vi "Begin.vi"(11 "Image Size":T1=enum."160x120") -> (0 "error out":errorcluster)   [LabVIEW 2011]
doc: "Called before other user functions, this VI is expected to open initial I/O refnums, load in file data, and do all program initialization. Notice that the <B>error out</B> terminal is simply used for data flow. Wiring it to other structures or subVIs ensures that this VI runs first."
uses:
  <vilib>/Rock Robotics/WPI/Camera/WPI_CameraImageSize.ctl
  <vilib>/Rock Robotics/WPI/Camera/WPI_CameraWhite Balance Values.ctl
  <vilib>/Rock Robotics/WPI/Camera/WPI_CameraExposure Values.ctl
  <vilib>/Rock Robotics/WPI/Camera/WPI_CameraFrameRate.ctl
  <vilib>/Rock Robotics/SystemInterfaces/DIO/FPGA_DIOPWMChannel.ctl
  <vilib>/Rock Robotics/SystemInterfaces/Typedef/FPGA_TypedefDigitalModule.ctl
  <vilib>/Rock Robotics/SystemInterfaces/Typedef/FPGA_TypedefAnalogModule.ctl
  <vilib>/Rock Robotics/SystemInterfaces/AI/FPGA_AIChannel.ctl
  <vilib>/Rock Robotics/SystemInterfaces/DIO/FPGA_DIOChannel.ctl
  <vilib>/Rock Robotics/SystemInterfaces/DIO/FPGA_DIORelayChannel.ctl
  <vilib>/Rock Robotics/WPI/Joystick/WPI_JoystickDeviceEnum.ctl
  <vilib>/Rock Robotics/WPI/Relay/WPI_RelayDirection.ctl
  <vilib>/Rock Robotics/SystemInterfaces/Typedef/FPGA_TypedefSolenoidModule.ctl
  <vilib>/Rock Robotics/WPI/Solenoid/WPI_SolenoidChannel.ctl
  <vilib>/Rock Robotics/WPI/RobotDrive/WPI_RobotDriveOpen4MotorWithVictor.vi
  <vilib>/Rock Robotics/WPI/MotorControl/WPI_MotorControlOpen Victor.vi
  <vilib>/Rock Robotics/WPI/Counter/WPI_CounterDigitalInputToDigitalSource.vi
  <vilib>/Rock Robotics/WPI/Counter/WPI_CounterOpen Gear Tooth Sensor Mode.vi
  <vilib>/Rock Robotics/WPI/Solenoid/WPI_SolenoidOpenDouble.vi
  <vilib>/Rock Robotics/WPI/Compressor/WPI_CompressorGetSetRefNum.vi
  <vilib>/Rock Robotics/WPI/Encoder/WPI_EncoderType.ctl
panel:
  in  "Image Size 2":T1=enum."160x120"
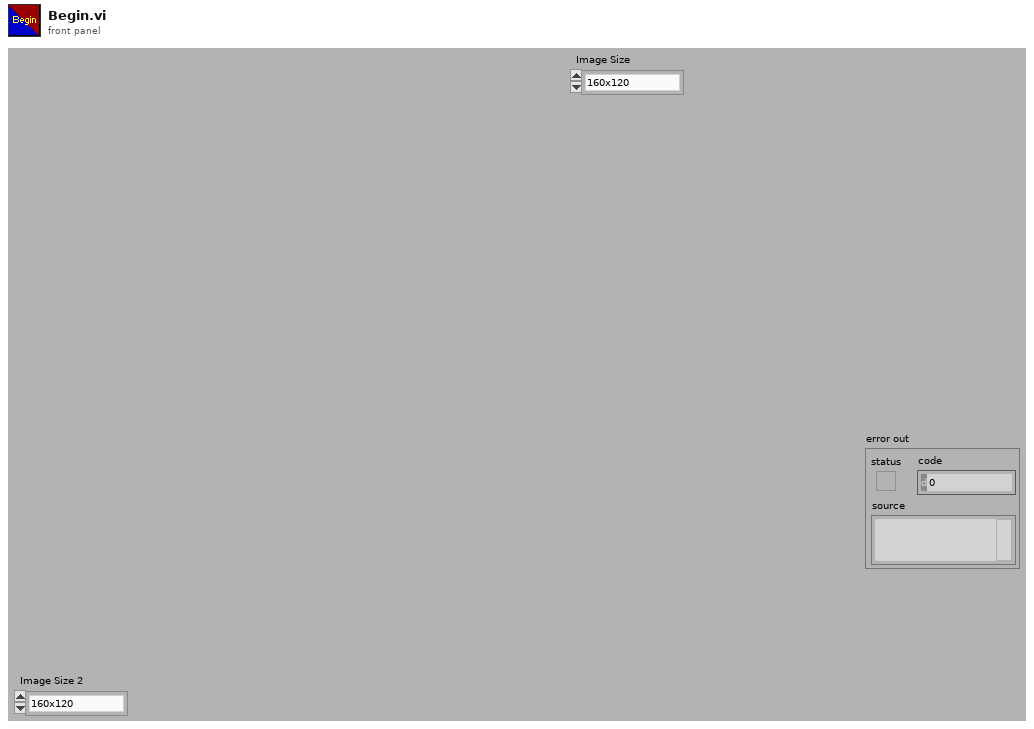
[diagram p1: front panel]
types:
  T1 = typedef "WPI_CameraImageSize.ctl" = enum16{"640x480", "320x240", "160x120"}
  T2 = typedef "FPGA_DIOChannel.ctl" = enum8{"DIO 1", "DIO 2", "DIO 3", "DIO 4", "DIO 5", "DIO 6", "DIO 7", "DIO 8", "DIO 9", "DIO 10", "DIO 11", "DIO 12", "DIO 13", "DIO 14", "Invalid"}
  T3 = typedef "FPGA_TypedefDigitalModule.ctl" = enum16{"Digital Module 1", "Digital Module 2"}
  T4 = typedef "WPI_SolenoidChannel.ctl" = enum8{"Solenoid 1", "Solenoid 2", "Solenoid 3", "Solenoid 4", "Solenoid 5", "Solenoid 6", "Solenoid 7", "Solenoid 8", "Invalid"}
  T5 = typedef "FPGA_TypedefSolenoidModule.ctl" = enum16{"Solenoid Module 1", "Solenoid Module 2"}
  T6 = typedef "WPI_RelayDirection.ctl" = enum16{"Both directions", "Forward only", "Reverse only"}
  T7 = typedef "FPGA_DIORelayChannel.ctl" = enum8{"Relay 1", "Relay 2", "Relay 3", "Relay 4", "Relay 5", "Relay 6", "Relay 7", "Relay 8", "Invalid"}
  T8 = typedef "WPI_JoystickDeviceEnum.ctl" = enum16{"USB 1", "USB 2", "USB 3", "USB 4", "Kinect 1", "Kinect 2"}
  T9 = typedef "FPGA_DIOPWMChannel.ctl" = enum8{"PWM 1", "PWM 2", "PWM 3", "PWM 4", "PWM 5", "PWM 6", "PWM 7", "PWM 8", "PWM 9", "PWM 10", "Invalid"}
  T10 = typedef "FPGA_AIChannel.ctl" = enum8{"AI 1", "AI 2", "AI 3", "AI 4", "AI 5", "AI 6", "AI 7", "AI 8", "Invalid"}
  T11 = typedef "FPGA_TypedefAnalogModule.ctl" = enum16{"Analog Module 1", "Analog Module 2"}
  T12 = typedef "WPI_CameraFrameRate.ctl" = u32
  T13 = typedef "WPI_CameraExposure Values.ctl" = enum16{"Auto", "Flicker-free 50 Hz", "Flicker-free 60 Hz", "Hold current"}
  T14 = typedef "WPI_CameraWhite Balance Values.ctl" = enum16{"Auto", "Fixed indoor", "Fixed outdoor 1", "Fixed outdoor 2", "Fixed fluorescent 1", "Fixed fluorescent 2", "Hold current"}
  T15 = typedef "WPI_MotorControlDeviceRef.ctl" = cluster{"DeviceStatus":errorcluster, "Type":enum16{"PWM", "CAN"}, "PWM":cluster{"Digital Module":T3, "PWM Channel":T9, "DeadBand":T16}, "CAN":cluster{"Device Number":u8, "Control Mode":T17, "Semaphore":T18, "Max Vout":dbl}, "Invert":bool, "TransformRef":T19, "InvTransformRef":T19}
  T16 = typedef "WPI_PWMDeadband.ctl" = cluster{"Name":string, "maxPositivePwm":i32, "minPositivePwm":i32, "centerPwm":i32, "maxNegativePwm":i32, "minNegativePwm":i32, "angularRange":u16}
  T17 = typedef "WPI_CANJaguar_ControlMode.ctl" = enum8{"Percent VBus", "Current", "Speed", "Position", "Voltage"}
  T18 = typedef "Semaphore RefNum" = refnum<k1>
  T19 = typedef "WPI_PWMTransform_ConPane.ctl" = refnum<vi>
  T20 = typedef "WPI_RobotDriveDevRef.ctl" = cluster{"DevStatus":errorcluster, "Motors[]":T15[], "Square Inputs":bool, "Max Output":dbl, "Isochronous":bool}
  T21 = typedef "WPI_CameraDevRef.ctl" = cluster{"Camera Address":string, "CameraStatus":errorcluster, "Acquire Image Notifier":refnum<notifier>}
  T22 = typedef "WPI_EncoderType.ctl" = enum16{"1x", "2x", "4x"}
  T23 = typedef "WPI_DigitalInputDevRef.ctl" = cluster{"DevStatus":errorcluster, "DIO Channel":T2, "Digital Module":T3}
  T24 = typedef "FPGA_CounterEncoderSourceConvertionLVSourceType.ctl" = cluster{"DevStatus":errorcluster, "AnalogTriggerMode?":bool, "DigitalMode":cluster{"Digital Module":T3, "DIO Channel":T25}, "AnalogTriggerMode":cluster{"AnalogTriggerIndex":T26, "OutputType":T27}}
  T25 = typedef "FPGA_DIODigitalSourceChannel.ctl" = enum8{"DIO 1", "DIO 2", "DIO 3", "DIO 4", "DIO 5", "DIO 6", "DIO 7", "DIO 8", "DIO 9", "DIO 10", "DIO 11", "DIO 12", "DIO 13", "DIO 14", "Disabled"}
  T26 = typedef "FPGA_AnalogTriggerIndex.ctl" = enum8{"Trig 0", "Trig 1", "Trig 2", "Trig 3", "Trig 4", "Trig 5", "Trig 6", "Trig 7", "Invalid"}
  T27 = typedef "FPGA_AnalogTriggerOutType.ctl" = enum16{"InWindow", "TriggerState", "Rising", "Falling"}
  T28 = typedef "WPI_EncoderDevRef.ctl" = cluster{"DevStatus":errorcluster, "EncoderIndex":T29, "CounterIndex":T30, "DistancePerCount":dbl, "Decoding Type":T22}
  T29 = typedef "FPGA_EncoderIdx.ctl" = enum8{"Enc 0", "Enc 1", "Enc 2", "Enc 3", "Invalid"}
  T30 = typedef "FPGA_CounterCtrSystemIndex.ctl" = enum8{"Ctr 0", "Ctr 1", "Ctr 2", "Ctr 3", "Ctr 4", "Ctr 5", "Ctr 6", "Ctr 7", "Invalid"}
  T31 = typedef "WPI_JoystickDevRef.ctl" = cluster{"Device":T8}
  T32 = typedef "WPI_AnalogChannelDevRef.ctl" = cluster{"DevStatus":errorcluster, "Analog Module":T11, "Analog Channel":T10}
  T33 = typedef "WPI_RelayDevRef.ctl" = cluster{"DevStatus":errorcluster, "Relay Channel":T7, "Digital Module":T3, "Relay Direction":T6}
  T34 = typedef "WPI_SolenoidDevRef.ctl" = cluster{"DevStatus":errorcluster, "Solenoid Module":T5, "Forward Solenoid Channel":T4, "Reverse Solenoid Channel":T4}
  T35 = typedef "WPI_CompressorDevRef.ctl" = cluster{"DevStatus":errorcluster, "DigitalInputDevRef":T23, "RelayDevRef":T33}
  T36 = typedef "WPI_CounterDevRef.ctl" = cluster{"DevStatus":errorcluster, "CntIndex":T30}
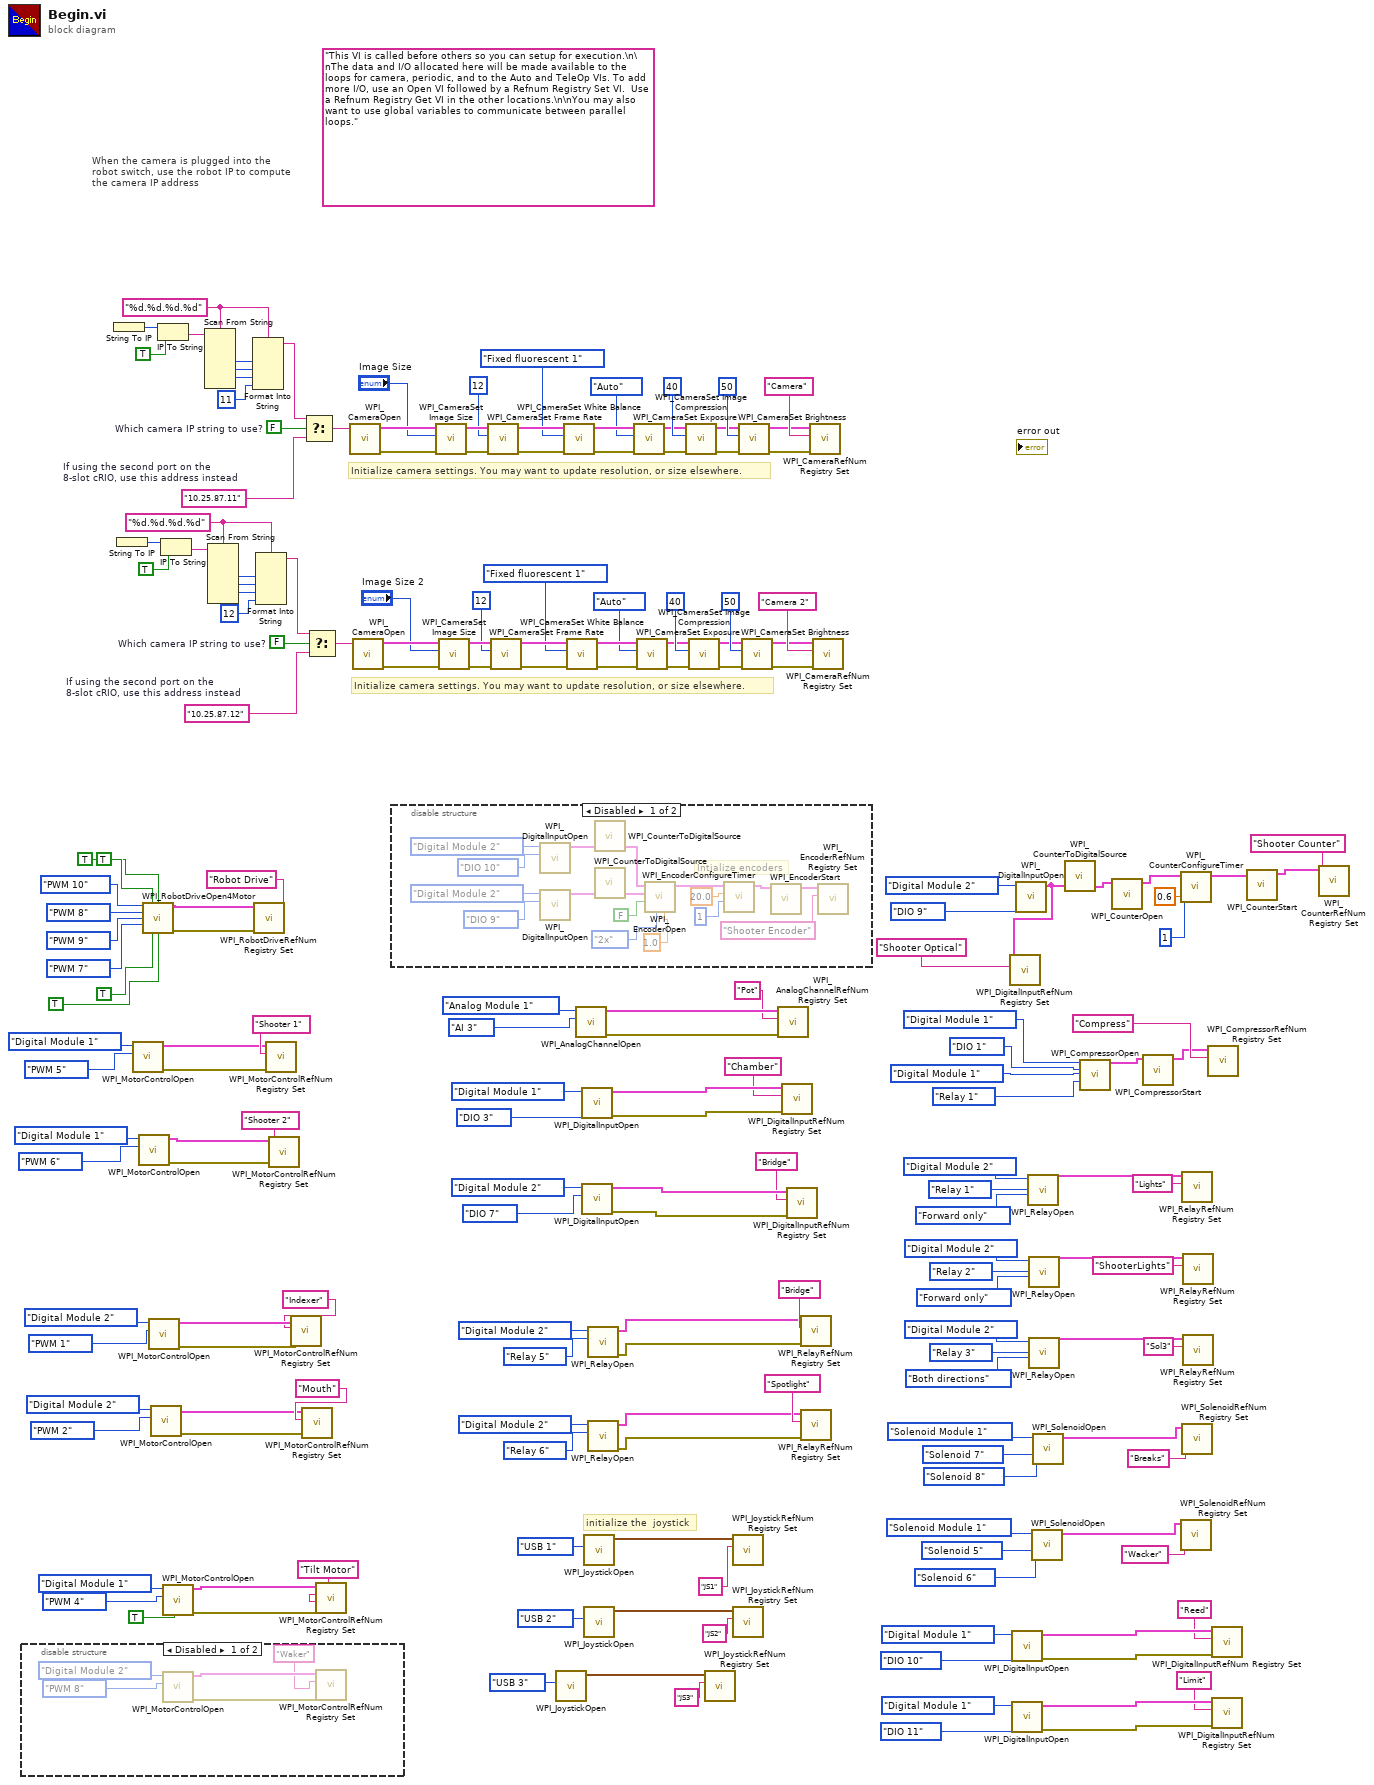
[diagram p0: block diagram]
diagram:
  w125 = FALSE  # Which camera IP string to use?
  w129 = "%d.%d.%d.%d" ("format string")
  w126 = "10.25.87.12"  # If using the second port on the 8-slot cRIO, use this address instead
  w158 = FALSE  # Which camera IP string to use?
  w162 = "%d.%d.%d.%d" ("format string")
  (unwired) "This VI is called before others so you can setup for execution.\n\nThe data and I/O allocated here will be made available to the loops for camera, periodic, and to the Auto and TeleOp VIs. To add more I/O, use an Open VI followed by a Refnum Registry Set VI.  Use a Refnum Registry Get VI in the other locations.\n\nYou may also want to use global variables to communicate between parallel loops."
  w159 = "10.25.87.11"  # If using the second port on the 8-slot cRIO, use this address instead
  # "initialize the  joystick"
  # "Initialize camera settings. You may want to update resolution, or size elsewhere."
  # "When the camera is plugged into the\nrobot switch, use the robot IP to compute\nthe camera IP address"
  # "Initialize camera settings. You may want to update resolution, or size elsewhere."
  n1 = disable-structure shown="Disabled" {
    frame Disabled {
      n2 = call-poly <vilib>:"WPI_MotorControlOpen.vi"("PWM Channel"=FPGA_DIOPWMChannel."PWM 8", "Digital Module (Module 1)"=FPGA_TypedefDigitalModule."Digital Module 2") -> ("error out"=w195:errorcluster, "MotorControlDeviceRef"=w194:T15)  [unwired: 8 in]
      n3 = call <vilib>:"WPI_MotorControlRefNum Registry Set.vi"("error in (no error)"=w195, "refnum name"="Waker", "MotorControlDevRef"=w194) -> ()  [unwired: 7 in, 2 out]
    }
    frame Enabled {
    }
  }
  n4 = String To IP() -> (0:w169:u32)  [unwired: 1 in]
  n5 = String To IP() -> (0:w136:u32)  [unwired: 1 in]
  n6 = call-poly <vilib>:"WPI_MotorControlOpen.vi"("PWM Channel"=FPGA_DIOPWMChannel."PWM 5", "Digital Module (Module 1)"=FPGA_TypedefDigitalModule."Digital Module 1") -> ("error out"=w108:errorcluster, "MotorControlDeviceRef"=w109:T15)  [unwired: 8 in]
  n7 = call-poly <vilib>:"WPI_MotorControlOpen.vi"("PWM Channel"=FPGA_DIOPWMChannel."PWM 6", "Digital Module (Module 1)"=FPGA_TypedefDigitalModule."Digital Module 1") -> ("error out"=w106:errorcluster, "MotorControlDeviceRef"=w107:T15)  [unwired: 8 in]
  n8 = call-poly <vilib>:"WPI_RobotDriveOpen4Motor.vi"("Rear Left Motor"=FPGA_DIOPWMChannel."PWM 10", "Rear Left Motor Inverted"=TRUE, "Rear Right Motor Inverted"=TRUE, "Rear Right Motor"=FPGA_DIOPWMChannel."PWM 8", "Front Left Motor"=FPGA_DIOPWMChannel."PWM 9", "Front Right Motor"=FPGA_DIOPWMChannel."PWM 7", "Front Left Motor Inverted"=TRUE, "Front Right Motor Inverted"=TRUE) -> ("RobotDriveDevRef"=w68:T20, "error out"=w67:errorcluster)  [unwired: 6 in]
  n9 = call-poly <vilib>:"WPI_MotorControlOpen.vi"("PWM Channel"=FPGA_DIOPWMChannel."PWM 1", "Digital Module (Module 1)"=FPGA_TypedefDigitalModule."Digital Module 2") -> ("error out"=w76:errorcluster, "MotorControlDeviceRef"=w77:T15)  [unwired: 8 in]
  n10 = call-poly <vilib>:"WPI_MotorControlOpen.vi"("PWM Channel"=FPGA_DIOPWMChannel."PWM 2", "Digital Module (Module 1)"=FPGA_TypedefDigitalModule."Digital Module 2") -> ("error out"=w101:errorcluster, "MotorControlDeviceRef"=w102:T15)  [unwired: 8 in]
  n11 = IP To String(1:TRUE ("dot notation? (F)"), 2:w169) -> (0:w167:string)
  n12 = IP To String(1:TRUE ("dot notation? (F)"), 2:w136) -> (0:w134:string)
  n13 = call-poly <vilib>:"WPI_MotorControlOpen.vi"("Invert"=TRUE, "PWM Channel"=FPGA_DIOPWMChannel."PWM 4", "Digital Module (Module 1)"=FPGA_TypedefDigitalModule."Digital Module 1") -> ("error out"=w95:errorcluster, "MotorControlDeviceRef"=w96:T15)  [unwired: 7 in]
  n14 = Scan From String(format string=w162, input string=w167) -> (output 1=w166:i32, output 2=w165:i32, output 3=w164:i32)  [unwired: 7 in, 3 out]
  n15 = Scan From String(format string=w129, input string=w134) -> (output 1=w133:i32, output 2=w132:i32, output 3=w131:i32)  [unwired: 7 in, 3 out]
  n16 = Format Into String(format string=w162, w166, w165, w164, 11 ("Compression")) -> (resulting string=w160:string)  [unwired: 2 in, 1 out]
  n17 = call <vilib>:"WPI_RobotDriveRefNum Registry Set.vi"("error in (no error)"=w67, "refnum name"="Robot Drive", "RobotDriveDevRef"=w68) -> ()  [unwired: 7 in, 2 out]
  n18 = Format Into String(format string=w129, w133, w132, w131, 12 ("Compression")) -> (resulting string=w127:string)  [unwired: 2 in, 1 out]
  n19 = call <vilib>:"WPI_MotorControlRefNum Registry Set.vi"("error in (no error)"=w108, "refnum name"="Shooter 1", "MotorControlDevRef"=w109) -> ()  [unwired: 7 in, 2 out]
  n20 = call <vilib>:"WPI_MotorControlRefNum Registry Set.vi"("error in (no error)"=w106, "refnum name"="Shooter 2", "MotorControlDevRef"=w107) -> ()  [unwired: 7 in, 2 out]
  n21 = call <vilib>:"WPI_MotorControlRefNum Registry Set.vi"("error in (no error)"=w76, "refnum name"="Indexer", "MotorControlDevRef"=w77) -> ()  [unwired: 7 in, 2 out]
  n22 = call <vilib>:"WPI_MotorControlRefNum Registry Set.vi"("error in (no error)"=w101, "refnum name"="Mouth", "MotorControlDevRef"=w102) -> ()  [unwired: 7 in, 2 out]
  n23 = Select(t=w160, s=w158, f=w159) -> (s? t:f=w161:string)
  n24 = Select(t=w127, s=w125, f=w126) -> (s? t:f=w128:string)
  n25 = call <vilib>:"WPI_MotorControlRefNum Registry Set.vi"("error in (no error)"=w95, "refnum name"="Tilt Motor", "MotorControlDevRef"=w96) -> ()  [unwired: 7 in, 2 out]
  n26 = call <vilib>:"WPI_CameraOpen.vi"("Camera Address"=w161) -> ("error out"=w181:errorcluster, "CameraDevRef"=w182:T21)  [unwired: 1 in, 8 out]
  n27 = call <vilib>:"WPI_CameraOpen.vi"("Camera Address"=w128) -> ("error out"=w148:errorcluster, "CameraDevRef"=w149:T21)  [unwired: 1 in, 8 out]
  n28 = disable-structure shown="Disabled" {
    frame Disabled {
      # "Intialize encoders"
      n29 = call <vilib>:"WPI_DigitalInputOpen.vi"("DIO Channel"=FPGA_DIOChannel."DIO 10", "Digital Module (Module 1)"=FPGA_TypedefDigitalModule."Digital Module 2") -> ("DigitalInputDevRef"=w210:T23)  [unwired: 8 in, 1 out]
      n30 = call <vilib>:"WPI_DigitalInputOpen.vi"("DIO Channel"=FPGA_DIOChannel."DIO 9", "Digital Module (Module 1)"=FPGA_TypedefDigitalModule."Digital Module 2") -> ("DigitalInputDevRef"=w206:T23)  [unwired: 8 in, 1 out]
      n31 = call-poly <vilib>:"WPI_CounterToDigitalSource.vi"("DigitalInputDevRef"=w210) -> ("Digital Source"=w209:T24)  [unwired: 6 in]
      n32 = call-poly <vilib>:"WPI_CounterToDigitalSource.vi"("DigitalInputDevRef"=w206) -> ("Digital Source"=w205:T24)  [unwired: 6 in]
      n33 = call <vilib>:"WPI_EncoderOpen.vi"("DistancePerCount"=1.0, "Decoding Type"=WPI_EncoderType."2x", "Invert Direction (False)"=FALSE, "BSource"=w205, "ASource"=w209) -> ("EncoderDevRef"=w203:T28)  [unwired: 5 in, 1 out]
      n34 = call <vilib>:"WPI_EncoderConfigureTimer.vi"("Number Samples to Average"=u8 1, "Minimum Rate"=20.0, "EncoderDevRef"=w203) -> ("EncoderDevRef"=w197:T28)  [unwired: 7 in, 1 out]
      n35 = call <vilib>:"WPI_EncoderStart.vi"("EncoderDevRef"=w197) -> ("EncoderDevRef"=w196:T28)  [unwired: 9 in, 1 out]
      n36 = call <vilib>:"WPI_EncoderRefNum Registry Set.vi"("refnum name"="Shooter Encoder", "EncoderDevRef"=w196) -> ()  [unwired: 8 in, 2 out]
    }
    frame Enabled {
    }
  }
  n37 = call <vilib>:"WPI_CameraSet Image Size.vi"("error in (no error)"=w181, "Image Size"="Image Size", "CameraDevRef"=w182) -> ("error out"=w180:errorcluster, "CameraDevRef Out"=w183:T21)  [unwired: 7 out]
  n38 = call <vilib>:"WPI_CameraSet Image Size.vi"("error in (no error)"=w148, "Image Size"="Image Size 2", "CameraDevRef"=w149) -> ("error out"=w147:errorcluster, "CameraDevRef Out"=w150:T21)  [unwired: 7 out]
  n39 = call <vilib>:"WPI_CameraSet Frame Rate.vi"("error in (no error)"=w180, "Frame Rate (fps)"=T12 12, "CameraDevRef"=w183) -> ("error out"=w179:errorcluster, "CameraDevRef Out"=w185:T21)  [unwired: 7 out]
  n40 = call <vilib>:"WPI_CameraSet Frame Rate.vi"("error in (no error)"=w147, "Frame Rate (fps)"=T12 12, "CameraDevRef"=w150) -> ("error out"=w146:errorcluster, "CameraDevRef Out"=w152:T21)  [unwired: 7 out]
  n41 = call <vilib>:"WPI_JoystickOpen.vi"("JoystickDevice"=WPI_JoystickDeviceEnum."USB 3") -> ("JoystickDevRef"=w45:T31)  [unwired: 10 out]
  n42 = call <vilib>:"WPI_CameraSet White Balance.vi"("error in (no error)"=w179, "White Balance"=WPI_CameraWhite_Balance_Values."Fixed fluorescent 1", "CameraDevRef"=w185) -> ("error out"=w178:errorcluster, "CameraDevRef Out"=w184:T21)  [unwired: 7 out]
  n43 = call <vilib>:"WPI_CameraSet White Balance.vi"("error in (no error)"=w146, "White Balance"=WPI_CameraWhite_Balance_Values."Fixed fluorescent 1", "CameraDevRef"=w152) -> ("error out"=w145:errorcluster, "CameraDevRef Out"=w151:T21)  [unwired: 7 out]
  n44 = call <vilib>:"WPI_AnalogChannelOpen.vi"("Analog Channel"=FPGA_AIChannel."AI 3", "Analog Module (Module 1)"=FPGA_TypedefAnalogModule."Analog Module 1") -> ("error out"=w90:errorcluster, "AIDeviceRef"=w92:T32)  [unwired: 8 in]
  n45 = call <vilib>:"WPI_DigitalInputOpen.vi"("DIO Channel"=FPGA_DIOChannel."DIO 3", "Digital Module (Module 1)"=FPGA_TypedefDigitalModule."Digital Module 1") -> ("error out"=w85:errorcluster, "DigitalInputDevRef"=w87:T23)  [unwired: 8 in]
  n46 = call <vilib>:"WPI_DigitalInputOpen.vi"("DIO Channel"=FPGA_DIOChannel."DIO 7", "Digital Module (Module 1)"=FPGA_TypedefDigitalModule."Digital Module 2") -> ("error out"=w57:errorcluster, "DigitalInputDevRef"=w59:T23)  [unwired: 8 in]
  n47 = call <vilib>:"WPI_JoystickOpen.vi"("JoystickDevice"=WPI_JoystickDeviceEnum."USB 1") -> ("JoystickDevRef"=w72:T31)  [unwired: 10 out]
  n48 = call <vilib>:"WPI_JoystickOpen.vi"("JoystickDevice"=WPI_JoystickDeviceEnum."USB 2") -> ("JoystickDevRef"=w71:T31)  [unwired: 10 out]
  n49 = call <vilib>:"WPI_RelayOpen.vi"("Relay Channel"=FPGA_DIORelayChannel."Relay 5", "Digital Module (Module 1)"=FPGA_TypedefDigitalModule."Digital Module 2") -> ("error out"=w62:errorcluster, "RelayDevRef"=w63:T33)  [unwired: 8 in]
  n50 = call <vilib>:"WPI_RelayOpen.vi"("Relay Channel"=FPGA_DIORelayChannel."Relay 6", "Digital Module (Module 1)"=FPGA_TypedefDigitalModule."Digital Module 2") -> ("error out"=w80:errorcluster, "RelayDevRef"=w81:T33)  [unwired: 8 in]
  n51 = call <vilib>:"WPI_CameraSet Exposure.vi"("error in (no error)"=w178, "Exposure"=WPI_CameraExposure_Values."Auto", "CameraDevRef"=w184) -> ("error out"=w177:errorcluster, "CameraDevRef Out"=w187:T21)  [unwired: 7 out]
  n52 = call <vilib>:"WPI_CameraSet Exposure.vi"("error in (no error)"=w145, "Exposure"=WPI_CameraExposure_Values."Auto", "CameraDevRef"=w151) -> ("error out"=w144:errorcluster, "CameraDevRef Out"=w154:T21)  [unwired: 7 out]
  n53 = call <vilib>:"WPI_CameraSet Image Compression.vi"("error in (no error)"=w177, "Compression"=40, "CameraDevRef"=w187) -> ("error out"=w176:errorcluster, "CameraDevRef Out"=w186:T21)  [unwired: 7 out]
  n54 = call <vilib>:"WPI_CameraSet Image Compression.vi"("error in (no error)"=w144, "Compression"=40, "CameraDevRef"=w154) -> ("error out"=w143:errorcluster, "CameraDevRef Out"=w153:T21)  [unwired: 7 out]
  n55 = call <vilib>:"WPI_JoystickRefNum Registry Set.vi"("refnum name"="JS3", "JoystickDevRef"=w45) -> ()  [unwired: 1 in, 9 out]
  n56 = call <vilib>:"WPI_JoystickRefNum Registry Set.vi"("refnum name"="JS1", "JoystickDevRef"=w72) -> ()  [unwired: 1 in, 9 out]
  n57 = call <vilib>:"WPI_JoystickRefNum Registry Set.vi"("refnum name"="JS2", "JoystickDevRef"=w71) -> ()  [unwired: 1 in, 9 out]
  n58 = call <vilib>:"WPI_CameraSet Brightness.vi"("error in (no error)"=w176, "Brightness"=50, "CameraDevRef"=w186) -> ("error out"=w174:errorcluster, "CameraDevRef Out"=w175:T21)  [unwired: 7 out]
  n59 = call <vilib>:"WPI_CameraSet Brightness.vi"("error in (no error)"=w143, "Brightness"=50, "CameraDevRef"=w153) -> ("error out"=w141:errorcluster, "CameraDevRef Out"=w142:T21)  [unwired: 7 out]
  n60 = call <vilib>:"WPI_AnalogChannelRefNum Registry Set.vi"("error in (no error)"=w90, "refnum name"="Pot", "AIDeviceRef"=w92) -> ()  [unwired: 7 in, 2 out]
  n61 = call <vilib>:"WPI_DigitalInputRefNum Registry Set.vi"("error in (no error)"=w85, "refnum name"="Chamber", "DigitalInputDevRef"=w87) -> ()  [unwired: 7 in, 2 out]
  n62 = call <vilib>:"WPI_DigitalInputRefNum Registry Set.vi"("error in (no error)"=w57, "refnum name"="Bridge", "DigitalInputDevRef"=w59) -> ()  [unwired: 7 in, 2 out]
  n63 = call <vilib>:"WPI_RelayRefNum Registry Set.vi"("error in (no error)"=w62, "refnum name"="Bridge", "RelayDevRef"=w63) -> ()  [unwired: 7 in, 2 out]
  n64 = call <vilib>:"WPI_RelayRefNum Registry Set.vi"("error in (no error)"=w80, "refnum name"="Spotlight", "RelayDevRef"=w81) -> ()  [unwired: 7 in, 2 out]
  n65 = call <vilib>:"WPI_CameraRefNum Registry Set.vi"("error in (no error)"=w174, "refnum name"="Camera", "CameraDevRef"=w175) -> ()  [unwired: 9 out]
  n66 = call <vilib>:"WPI_CameraRefNum Registry Set.vi"("error in (no error)"=w141, "refnum name"="Camera 2", "CameraDevRef"=w142) -> ()  [unwired: 9 out]
  n67 = call <vilib>:"WPI_DigitalInputOpen.vi"("DIO Channel"=FPGA_DIOChannel."DIO 10", "Digital Module (Module 1)"=FPGA_TypedefDigitalModule."Digital Module 1") -> ("error out"=w6:errorcluster, "DigitalInputDevRef"=w8:T23)  [unwired: 8 in]
  n68 = call <vilib>:"WPI_DigitalInputOpen.vi"("DIO Channel"=FPGA_DIOChannel."DIO 11", "Digital Module (Module 1)"=FPGA_TypedefDigitalModule."Digital Module 1") -> ("error out"=w1:errorcluster, "DigitalInputDevRef"=w3:T23)  [unwired: 8 in]
  n69 = call <vilib>:"WPI_DigitalInputOpen.vi"("DIO Channel"=FPGA_DIOChannel."DIO 9", "Digital Module (Module 1)"=FPGA_TypedefDigitalModule."Digital Module 2") -> ("DigitalInputDevRef"=w53:T23)  [unwired: 8 in, 1 out]
  n70 = call <vilib>:"WPI_DigitalInputRefNum Registry Set.vi"("refnum name"="Shooter Optical", "DigitalInputDevRef"=w53) -> ()  [unwired: 8 in, 2 out]
  n71 = call <vilib>:"WPI_RelayOpen.vi"("Relay Direction"=WPI_RelayDirection."Forward only", "Relay Channel"=FPGA_DIORelayChannel."Relay 1", "Digital Module (Module 1)"=FPGA_TypedefDigitalModule."Digital Module 2") -> ("RelayDevRef"=w37:T33)  [unwired: 7 in, 1 out]
  n72 = call <vilib>:"WPI_RelayOpen.vi"("Relay Direction"=WPI_RelayDirection."Forward only", "Relay Channel"=FPGA_DIORelayChannel."Relay 2", "Digital Module (Module 1)"=FPGA_TypedefDigitalModule."Digital Module 2") -> ("RelayDevRef"=w32:T33)  [unwired: 7 in, 1 out]
  n73 = call <vilib>:"WPI_RelayOpen.vi"("Relay Direction"=WPI_RelayDirection."Both directions", "Relay Channel"=FPGA_DIORelayChannel."Relay 3", "Digital Module (Module 1)"=FPGA_TypedefDigitalModule."Digital Module 2") -> ("RelayDevRef"=w27:T33)  [unwired: 7 in, 1 out]
  n74 = call-poly <vilib>:"WPI_SolenoidOpen.vi"("Reverse Solenoid Channel"=WPI_SolenoidChannel."Solenoid 6", "Forward Solenoid Channel"=WPI_SolenoidChannel."Solenoid 5", "Solenoid Module (Module 1)"=FPGA_TypedefSolenoidModule."Solenoid Module 1") -> ("SolenoidDevRef"=w15:T34)  [unwired: 7 in, 1 out]
  n75 = call-poly <vilib>:"WPI_SolenoidOpen.vi"("Reverse Solenoid Channel"=WPI_SolenoidChannel."Solenoid 8", "Forward Solenoid Channel"=WPI_SolenoidChannel."Solenoid 7", "Solenoid Module (Module 1)"=FPGA_TypedefSolenoidModule."Solenoid Module 1") -> ("SolenoidDevRef"=w20:T34)  [unwired: 7 in, 1 out]
  n76 = call-poly <vilib>:"WPI_CounterToDigitalSource.vi"("DigitalInputDevRef"=w53) -> ("Digital Source"=w52:T24)  [unwired: 6 in]
  n77 = call <vilib>:"WPI_CompressorOpen.vi"("Pressure Switch Digital Module (Module 1)"=FPGA_TypedefDigitalModule."Digital Module 1", "Pressure Switch DIO Channel"=FPGA_DIOChannel."DIO 1", "Relay Digital Module (Module 1)"=FPGA_TypedefDigitalModule."Digital Module 1", "Relay Channel"=FPGA_DIORelayChannel."Relay 1") -> ("CompressorDevRef"=w11:T35)  [unwired: 10 in, 1 out]
  n78 = call-poly <vilib>:"WPI_CounterOpen.vi"("Source"=w52) -> ("CounterDevRef"=w48:T36)  [unwired: 9 in, 1 out]
  n79 = call <vilib>:"WPI_CompressorStart.vi"("CompressorDevRef"=w11) -> ("CompressorDevRef"=w12:T35)  [unwired: 9 in, 1 out]
  n80 = call <vilib>:"WPI_CounterConfigureTimer.vi"("Number Samples to Average"=u8 1, "MaxPeriod (sec)"=0.6, "CounterDevRef in"=w48) -> ("CounterDevRef out"=w50:T36)  [unwired: 7 in, 1 out]
  n81 = call <vilib>:"WPI_SolenoidRefNum Registry Set.vi"("refnum name"="Wacker", "SolenoidDevRef"=w15) -> ()  [unwired: 8 in, 2 out]
  n82 = call <vilib>:"WPI_RelayRefNum Registry Set.vi"("refnum name"="Lights", "RelayDevRef"=w37) -> ()  [unwired: 8 in, 2 out]
  n83 = call <vilib>:"WPI_SolenoidRefNum Registry Set.vi"("refnum name"="Breaks", "SolenoidDevRef"=w20) -> ()  [unwired: 8 in, 2 out]
  n84 = call <vilib>:"WPI_RelayRefNum Registry Set.vi"("refnum name"="ShooterLights", "RelayDevRef"=w32) -> ()  [unwired: 8 in, 2 out]
  n85 = call <vilib>:"WPI_RelayRefNum Registry Set.vi"("refnum name"="Sol3", "RelayDevRef"=w27) -> ()  [unwired: 8 in, 2 out]
  n86 = call <vilib>:"WPI_CompressorRefNum Registry Set.vi"("refnum name"="Compress", "CompressorDevRef"=w12) -> ()  [unwired: 8 in, 2 out]
  n87 = call <vilib>:"WPI_DigitalInputRefNum Registry Set.vi"("error in (no error)"=w6, "refnum name"="Reed", "DigitalInputDevRef"=w8) -> ()  [unwired: 7 in, 2 out]
  n88 = call <vilib>:"WPI_DigitalInputRefNum Registry Set.vi"("error in (no error)"=w1, "refnum name"="Limit", "DigitalInputDevRef"=w3) -> ()  [unwired: 7 in, 2 out]
  n89 = call <vilib>:"WPI_CounterStart.vi"("CounterDevRef in"=w50) -> ("CounterDevRef out"=w49:T36)  [unwired: 9 in, 1 out]
  n90 = call <vilib>:"WPI_CounterRefNum Registry Set.vi"("refnum name"="Shooter Counter", "CounterDevRef"=w49) -> ()  [unwired: 8 in, 2 out]
